vi "DB_EscribeTablaPolar.vi"(8 "error in (no error)":errorcluster, 9 "Polar_cluster":T1, 10 "Equipo_Medicion":T2={"ID_EQUIPO"=0, "IP_EQUIPO"="", "NOMBRE_EQUIPO"="", "ESTADO_EQUIPO"="", "DESCRIPCION"="", "ID_MEDICION"=0, "ESTADO_MEDICION"="", "TIEMPO_MEDICION"="12-02-2019 18:41"}, 11 "db in":T3) -> (0 "error out":errorcluster, 3 "db out":T3)   [LabVIEW 2018]
uses:
  <vilib>/addons/database/Connection.llb/Conn ObjectReference.ctl
  Controls/Equipos_Medicion_cluster.ctl
  Controls/Polar_cluster.ctl
  <vilib>/addons/database/Connection.llb/Conn Execute.vi
  <vilib>/addons/database/Recordset.llb/Rec Destroy - Connection.vi
  <vilib>/addons/database/NI_Database_API.lvlib
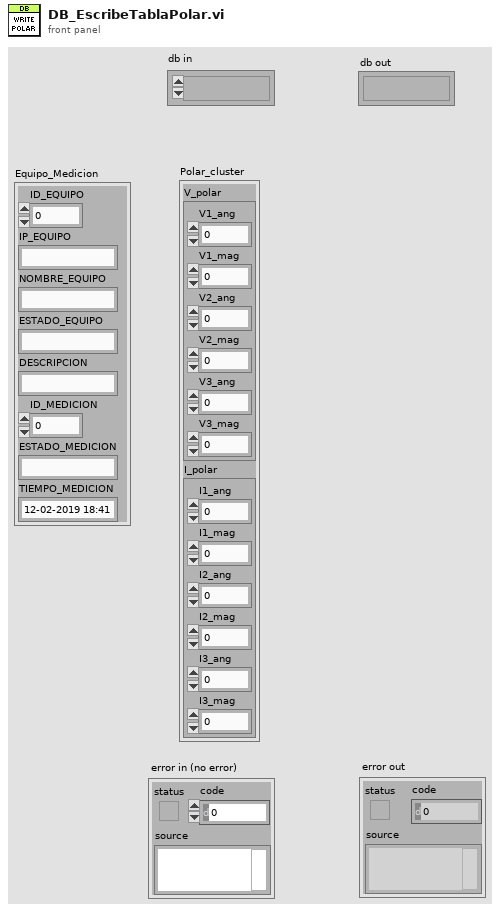
[diagram p1: front panel]
types:
  T1 = typedef "Polar_cluster.ctl" = cluster{"V_polar":cluster{"V1_ang":sgl, "V1_mag":sgl, "V2_ang":sgl, "V2_mag":sgl, "V3_ang":sgl, "V3_mag":sgl}, "I_polar":cluster{"I1_ang":sgl, "I1_mag":sgl, "I2_ang":sgl, "I2_mag":sgl, "I3_ang":sgl, "I3_mag":sgl}}
  T2 = typedef "Equipos_Medicion_cluster.ctl" = cluster{"ID_EQUIPO":i32, "IP_EQUIPO":string, "NOMBRE_EQUIPO":string, "ESTADO_EQUIPO":string, "DESCRIPCION":string, "ID_MEDICION":i32, "ESTADO_MEDICION":string, "TIEMPO_MEDICION":string}
  T3 = typedef "NI_Database_API.lvlib/Conn ObjectReference.ctl" = refnum<k1>
  T4 = cluster{"V1_ang":sgl, "V1_mag":sgl, "V2_ang":sgl, "V2_mag":sgl, "V3_ang":sgl, "V3_mag":sgl}
  T5 = cluster{"I1_ang":sgl, "I1_mag":sgl, "I2_ang":sgl, "I2_mag":sgl, "I3_ang":sgl, "I3_mag":sgl}
  T6 = typedef "NI_Database_API.lvlib/Rec ObjectReference.ctl" = refnum<k1>
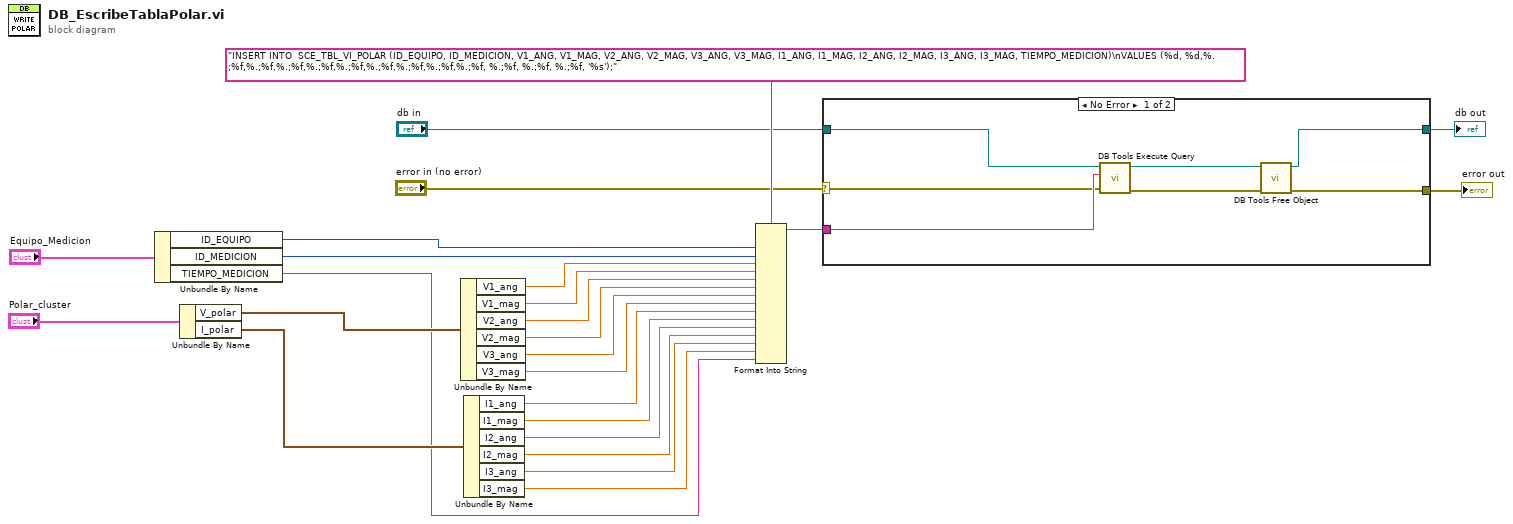
[diagram p0: block diagram]
diagram:
  n1 = Unbundle By Name("Equipo_Medicion") -> ("ID_EQUIPO"=w21:i32, "ID_MEDICION"=w20:i32, "TIEMPO_MEDICION"=w5:string)
  n2 = Unbundle By Name("Polar_cluster") -> ("V_polar"=w16:T4, "I_polar"=w15:T5)
  n3 = Unbundle By Name(w16) -> ("V1_ang"=w19:sgl, "V1_mag"=w18:sgl, "V2_ang"=w17:sgl, "V2_mag"=w14:sgl, "V3_ang"=w13:sgl, "V3_mag"=w12:sgl)
  n4 = Unbundle By Name(w15) -> ("I1_ang"=w11:sgl, "I1_mag"=w10:sgl, "I2_ang"=w9:sgl, "I2_mag"=w8:sgl, "I3_ang"=w7:sgl, "I3_mag"=w6:sgl)
  n5 = Format Into String(format string="INSERT INTO  SCE_TBL_VI_POLAR (ID_EQUIPO, ID_MEDICION, V1_ANG, V1_MAG, V2_ANG, V2_MAG, V3_ANG, V3_MAG, I1_ANG, I1_MAG, I2_ANG, I2_MAG, I3_ANG, I3_MAG, TIEMPO_MEDICION)\nVALUES (%d, %d,%.;%f,%.;%f,%.;%f,%.;%f,%.;%f,%.;%f,%.;%f,%.;%f,%.;%f, %.;%f, %.;%f, %.;%f, '%s');" ("SQL"), w21, w20, w19, w18, w17, w14, w13, w12, w11, w10, w9, w8, w7, w6, w5) -> (resulting string=w25:string)  [unwired: 2 in, 1 out]
  n6 = case shown="No Error" "error in (no error)" {
    selector: "error in (no error)" -> [w30 w34]
    tunnel: w25 -> [w31 _]
    tunnel: [w28 w34] -> w23
    tunnel: "db in" -> [w29 w33]
    tunnel: [w26 w33] -> w3
    frame No Error {
      n7 = call-poly <vilib>:"DB Tools Execute Query.vi"("error in (no error)"=w30, "SQL query"=w31, "connection reference"=w29) -> ("error out"=w32:errorcluster, "recordset reference"=w27:T6)  [unwired: 5 in]
      n8 = call-poly <vilib>:"DB Tools Free Object.vi"("error in (no error)"=w32, "recordset reference"=w27) -> ("error out"=w28:errorcluster, "connection reference"=w26:T3)  [unwired: 8 in]
    }
    frame Error {
    }
  }
  "error out" <- w23
  "db out" <- w3
